vi "subvi_load_image.vi"(0 "Path to single file (png or txt with metadata)":path) -> (1 "Paths to data":cluster{"Picture":path, "Text":path}, 2 "loaded picture":picture, 3 "Resolution [px]":i16[](array[numeric]), 4 "Stop":bool)   [LabVIEW 2016]
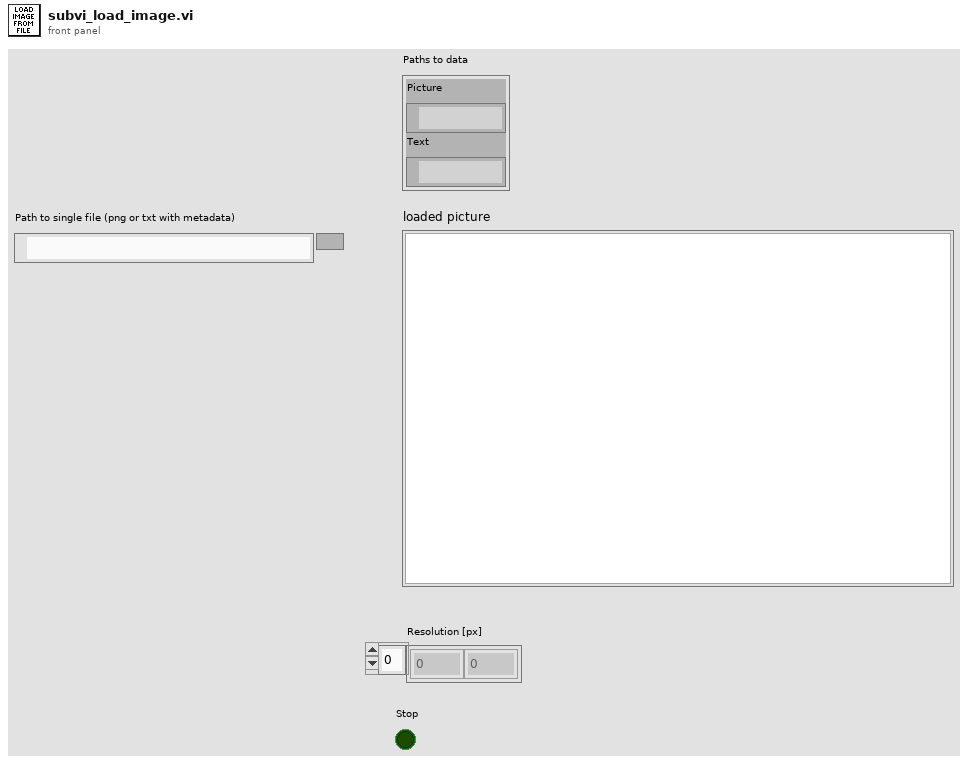
[diagram p1: front panel]
types:
  T1 = typedef "imagedata.ctl" = cluster{"image type":i32, "image depth":i32, "image":u8[], "mask":u8[], "colors":u32[], "Rectangle":cluster{"left":i16, "top":i16, "right":i16, "bottom":i16}}
  T2 = cluster{"left":i16, "top":i16, "right":i16, "bottom":i16}
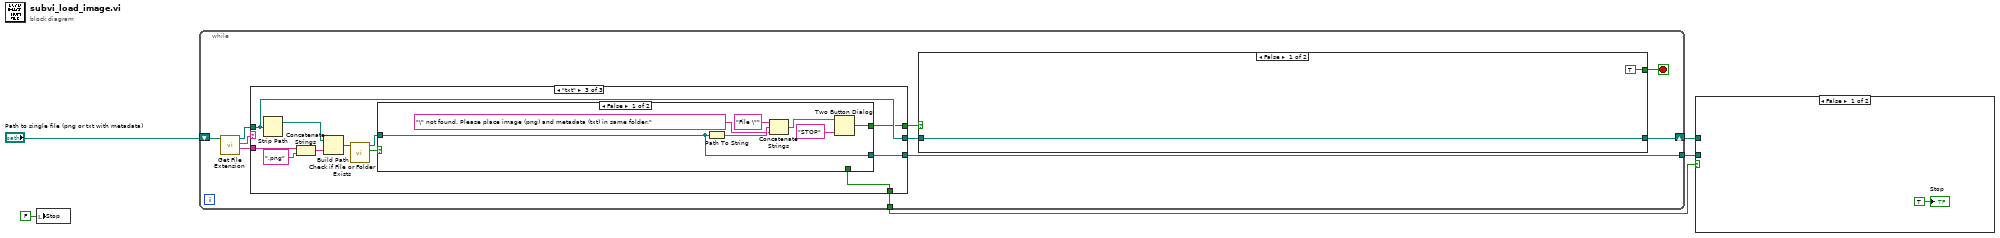
[diagram p0: block diagram]
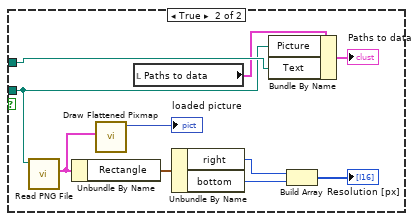
[diagram p2: hidden frame]
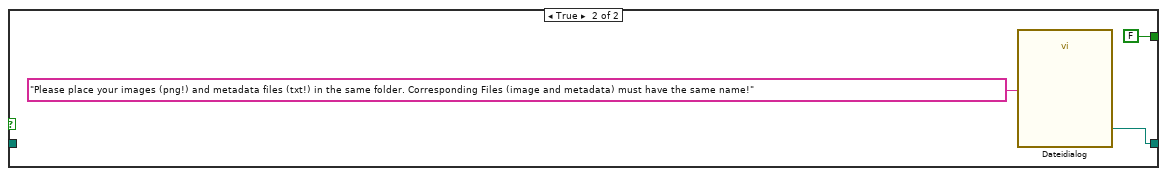
[diagram p3: hidden frame]
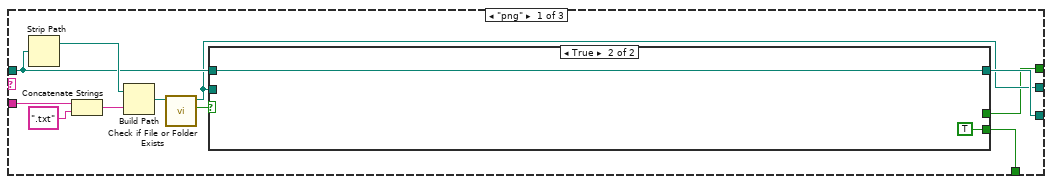
[diagram p4: hidden frame]
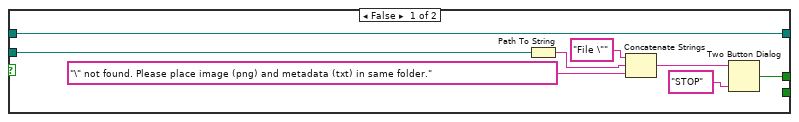
[diagram p5: hidden frame]
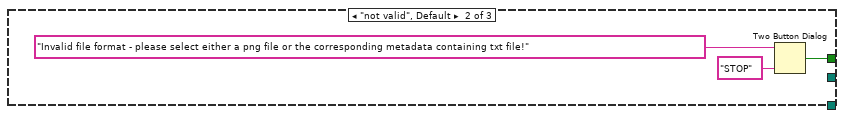
[diagram p6: hidden frame]
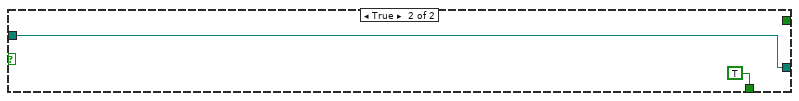
[diagram p7: hidden frame]
diagram:
  n1 = local write "Stop"(FALSE ("Stop")) -> ()
  n2 = while {
    tunnel: [w15] -> w4
    shift-right: [w8] -> w5
    shift-left: "Path to single file (png or txt with metadata)" -> [w14]
    tunnel: [w6] -> w2
    stop <- w9 stop-if-true
    n3 = call <vilib>:"Get File Extension.vi"("file"=w14) -> ("filename without extension"=w12:string, "lowercase file extension"=w13:string, "dup file"=w11:path)  [unwired: 6 in, 2 out]
    n4 = case shown="\"txt\"" w13 {
      tunnel: w12 -> [w28 _ w55]
      tunnel: w11 -> [w25 _ w47]
      tunnel: [w24 _ w49] -> w15
      tunnel: [w23 _ w47] -> w7
      tunnel: [w22 w42 w46] -> w10
      tunnel: [w21 _ w45] -> w6
      frame "png" {
        n5 = Strip Path(path=w25) -> (stripped path=w31:path)  [unwired: 1 out]
        n6 = Concatenate Strings(w28, ".txt" ("String")) -> (w29:string)
        n7 = Build Path(base path=w31, name or relative path=w29) -> (appended path=w27:path)
        n8 = call <vilib>:"Check if File or Folder Exists.vi"("path"=w27) -> ("file or folder exists?"=w26:bool, "dup path"=w23:path)  [unwired: 8 in, 1 out]
        n9 = case shown="True" w26 {
          tunnel: w23 -> [w38 _]
          tunnel: [w34 w41] -> w24
          tunnel: w25 -> [w34 w41]
          tunnel: [w32 _] -> w22
          tunnel: [_ TRUE] -> w21
          frame False {
            n10 = Path To String(path=w38) -> (string=w37:string)
            n11 = Concatenate Strings("File \"" ("String"), w37, "\" not found. Please place image (png) and metadata (txt) in same folder." ("String")) -> (w35:string)
            n12 = Two Button Dialog(message=w35, 1:"STOP" ("Text für F-Schaltfläche (\"Abbrechen\")")) -> (T button?=w32:bool)  [unwired: 1 in]
          }
          frame True {
          }
        }
      }
      frame "not valid", Default {
        n13 = Two Button Dialog(message="Invalid file format - please select either a png file or the corresponding metadata containing txt file!" ("Nachricht"), 1:"STOP" ("Text für F-Schaltfläche (\"Abbrechen\")")) -> (T button?=w42:bool)  [unwired: 1 in]
      }
      frame "txt" {
        n14 = Strip Path(path=w47) -> (stripped path=w48:path)  [unwired: 1 out]
        n15 = Concatenate Strings(w55, ".png" ("String")) -> (w53:string)
        n16 = Build Path(base path=w48, name or relative path=w53) -> (appended path=w50:path)
        n17 = call <vilib>:"Check if File or Folder Exists.vi"("path"=w50) -> ("file or folder exists?"=w52:bool, "dup path"=w51:path)  [unwired: 8 in, 1 out]
        n18 = case shown="False" w52 {
          tunnel: w51 -> [w58 w64]
          tunnel: [w58 w64] -> w49
          tunnel: [w56 _] -> w46
          tunnel: [_ TRUE] -> w45
          frame False {
            n19 = Path To String(path=w58) -> (string=w61:string)
            n20 = Concatenate Strings("File \"" ("String"), w61, "\" not found. Please place image (png) and metadata (txt) in same folder." ("String")) -> (w59:string)
            n21 = Two Button Dialog(message=w59, 1:"STOP" ("Text für F-Schaltfläche (\"Abbrechen\")")) -> (T button?=w56:bool)  [unwired: 1 in]
          }
          frame True {
          }
        }
      }
    }
    n22 = case shown="False" w10 {
      tunnel: [TRUE FALSE] -> w9
      tunnel: [w16 w18] -> w8
      tunnel: w7 -> [w16 _]
      frame False {
      }
      frame True {
        n23 = call "Dateidialog"("prompt"="Please place your images (png!) and metadata files (txt!) in the same folder. Corresponding Files (image and metadata) must have the same name!") -> ("selected path"=w18:path)  [unwired: 11 in, 3 out]
      }
    }
  }
  n24 = case shown="False" w2 {
    tunnel: w5 -> [_ w75]
    tunnel: w4 -> [_ w74]
    frame False {
      "Stop" <- TRUE ("Stop")
    }
    frame True {
      n25 = call <vilib>:"Read PNG File.vi"("path to PNG file"=w74) -> ("image data"=w69:T1)  [unwired: 8 in, 2 out]
      n26 = Unbundle By Name(w69) -> ("Rectangle"=w70:T2)
      n27 = call <vilib>:"Draw Flattened Pixmap.vi"("image data"=w69) -> ("new picture"=→"loaded picture":picture)  [unwired: 8 in]
      n28 = local read "Paths to data"() -> (w67:cluster{"Picture":path, "Text":path})
      n29 = Unbundle By Name(w70) -> ("right"=w71:i16, "bottom"=w73:i16)
      n30 = Bundle By Name(cluster=w67, "Picture"=w74, "Text"=w75) -> (→"Paths to data":cluster{"Picture":path, "Text":path})
      n31 = Build Array(w71, w73) -> (→"Resolution [px]":i16[])
    }
  }
